vi "Target Path.vi"(11 "Processing in":refnum<class "Processing.lvclass">) -> (3 "Processing out":refnum<class "Processing.lvclass">, 5 "Target Path":string)   [LabVIEW 2020, in "HTTP Server.lvlib" / "Processing.lvclass"]
uses:
  Processing.lvclass
  Processing.lvclass/Processing.ctl
  lv-http-util/HTTP Utils/Request/Request.lvclass
  lv-uri/URI/URI/URI.lvclass
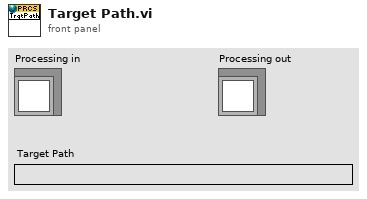
[diagram p1: front panel]
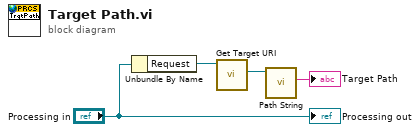
[diagram p0: block diagram]
diagram:
  n1 = Unbundle By Name("Processing in") -> ("Request"=w2:refnum<class "Request.lvclass">)
  n2 = call "Get Target URI.vi"("Request in"=w2) -> ("Target URI"=w4:refnum<class "URI.lvclass">)  [unwired: 8 in, 2 out]
  n3 = call "Path String.vi"("URI in"=w4) -> ("Path String"=→"Target Path":string)  [unwired: 9 in, 1 out]
  "Processing out" <- "Processing in"
